vi "String Cases.vi"() -> ()   [LabVIEW 2018]
panel:
  in  "String":string
  out "UPPER CASE":string
  out "Start case":string
  out "lower case":string
  out "Title Case":string
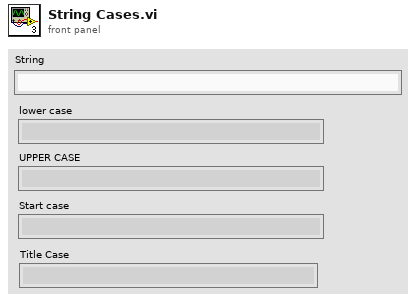
[diagram p1: front panel]
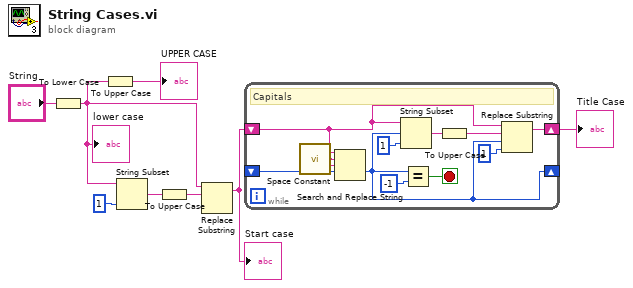
[diagram p0: block diagram]
diagram:
  n1 = To Lower Case(string="String") -> (all lower case string=w3:string)
  "lower case" <- w3
  n2 = To Upper Case(1:w3) -> (0:→"UPPER CASE":string)
  n3 = String Subset(string=w3, length (rest)=1 ("length (rest)")) -> (substring=w7:string)  [unwired: 1 in]
  n4 = To Upper Case(1:w7) -> (0:w6:string)
  n5 = Replace Substring(4:w6, 5:w3) -> (1:w4:string)  [unwired: 2 in, 1 out]
  "Start case" <- w4
  n6 = while {
    shift-right: [w13] -> w5
    shift-left: w4 -> [w15]
    shift-right: [w11] -> _
    shift-left: _ -> [w12]
    stop <- w9 stop-if-true
    # "Capitals"
    n7 = call <vilib>:"Space Constant.vi"() -> ("String"=w19:string)
    n8 = Search and Replace String(input string=w15, search string=w19, replace string=w19, offset=w12) -> (offset past replacement=w11:i32)  [unwired: 4 in, 3 out]
    n9 = String Subset(string=w15, offset (0)=w11, length (rest)=1 ("length (rest)")) -> (substring=w17:string)
    n10 = Equal?(x=w11, y=-1) -> (x = y?=w9:bool)
    n11 = To Upper Case(1:w17) -> (0:w16:string)
    n12 = Replace Substring(2:1 ("length (len. of substring)"), 3:w11, 4:w16, 5:w15) -> (1:w13:string)  [unwired: 1 out]
  }
  "Title Case" <- w5
